vi "GetInstance.vi"(0 "Error Logger in":refnum<class "Error Logger.lvclass">, 11 "error in (no error)":errorcluster, 13 "Get[T]\\Set[F]":bool=TRUE) -> (4 "Error Logger out":refnum<class "Error Logger.lvclass">, 15 "error out":errorcluster)   [LabVIEW 2014, in "Error Logger.lvclass"]
uses:
  Error Logger.lvclass
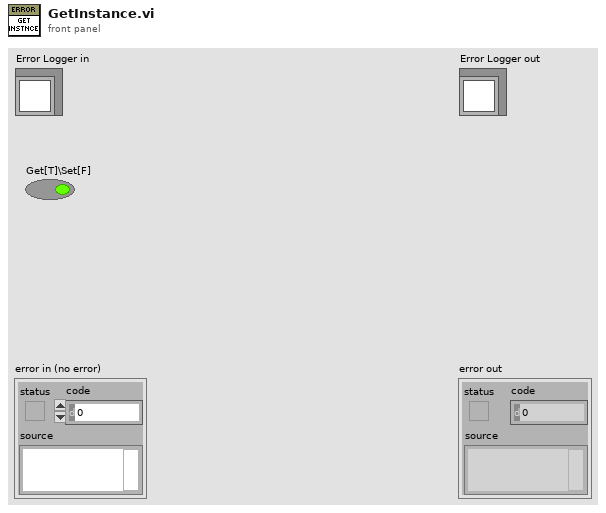
[diagram p1: front panel]
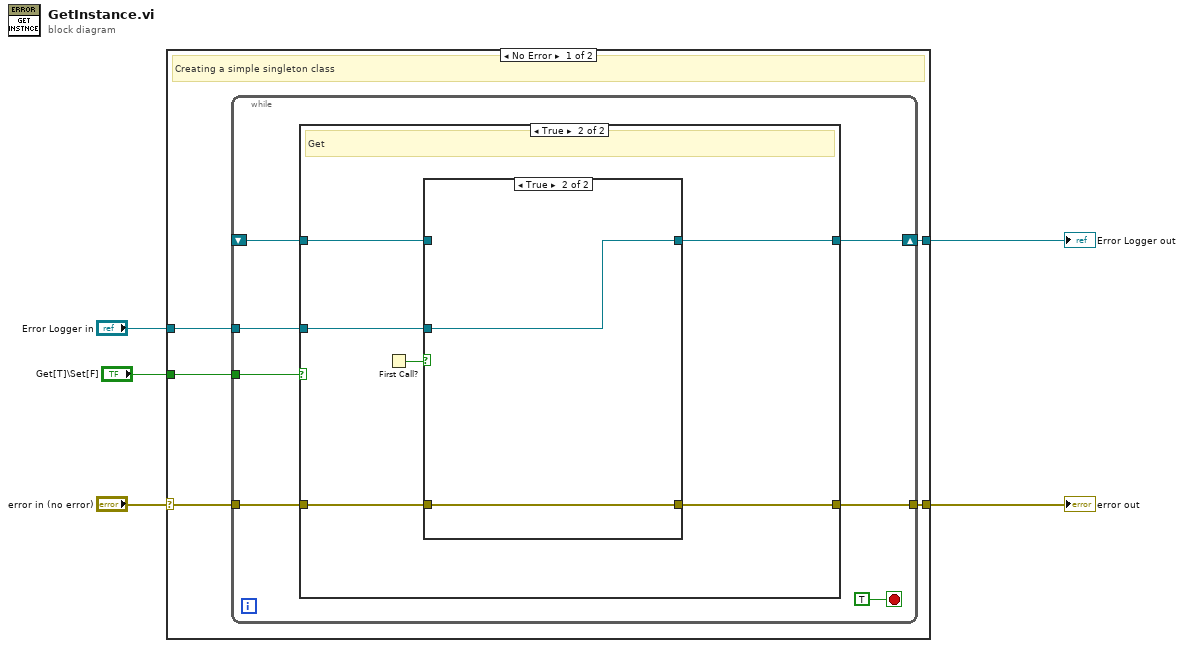
[diagram p0: block diagram]
diagram:
  n1 = case shown="No Error" "error in (no error)" {
    selector: "error in (no error)" -> [w7 w31]
    tunnel: [w8 w31] -> w4
    tunnel: [w9 w30] -> w2
    tunnel: "Error Logger in" -> [w10 w30]
    tunnel: "Get[T]\\Set[F]" -> [w6 _]
    frame No Error {
      # "Creating a simple singleton class"
      n2 = while {
        tunnel: w10 -> [w15]
        shift-right: [w16] -> w9
        shift-left: _ -> [w14]
        tunnel: [w13] -> w8
        tunnel: w7 -> [w12]
        tunnel: w6 -> [w11]
        stop <- TRUE stop-if-true
        n3 = case shown="True" w11 {
          tunnel: [w19 w24] -> w16
          tunnel: w15 -> [w19 w23]
          tunnel: w14 -> [_ w22]
          tunnel: [w18 w21] -> w13
          tunnel: w12 -> [w18 w20]
          frame False {
            # "Set"
          }
          frame True {
            # "Get"
            n4 = First Call?() -> (First Call?: T/F=w25:bool)
            n5 = case shown="True" w25 {
              tunnel: [w27 w29] -> w24
              tunnel: w23 -> [_ w29]
              tunnel: w22 -> [w27 _]
              tunnel: [w26 w28] -> w21
              tunnel: w20 -> [w26 w28]
              frame False {
              }
              frame True {
              }
            }
          }
        }
      }
    }
    frame Error {
    }
  }
  "error out" <- w4
  "Error Logger out" <- w2
